vi "Generate String.vi"(8 "error in (no error)":errorcluster, 11 "object in":refnum<class "CodeElement.lvclass">) -> (0 "error out":errorcluster, 2 "String":string, 3 "object out":refnum<class "CodeElement.lvclass">)   [LabVIEW 2017, in "CodeElement.lvclass"]
uses:
  CodeElement.lvclass
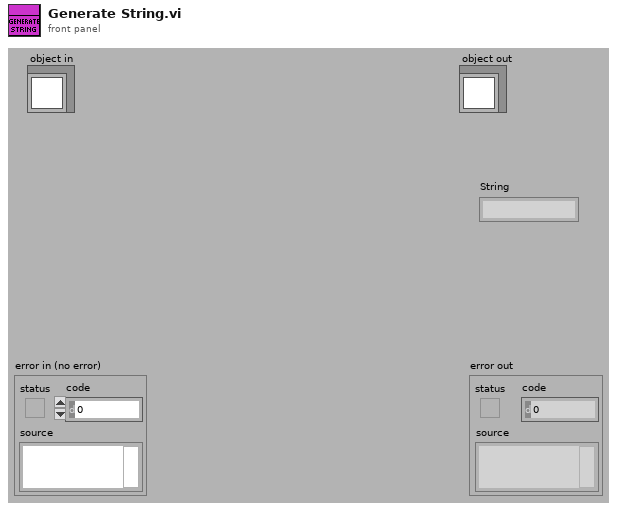
[diagram p1: front panel]
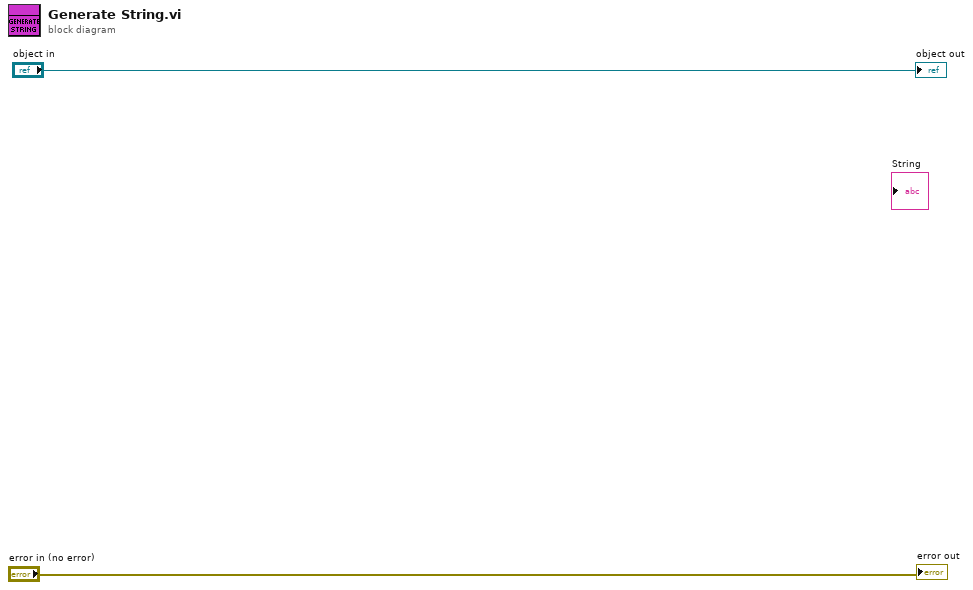
[diagram p0: block diagram]
diagram:
  "error out" <- "error in (no error)"
  "object out" <- "object in"
